vi "Example - Creating and Building an Installer.vi"() -> ()   [LabVIEW 2020]
doc: "Demonstrates the use of the Installer Builder API to create and build an Installer build specification."
uses:
  <vilib>/InstallerBuilder/Classes/Win_Installer/Product Version.ctl
  <vilib>/InstallerBuilder/Classes/Win_Installer/AB_Win_Installer.lvclass/AB_Win_Installer.ctl
  <vilib>/InstallerBuilder/Classes/Win_Source/AB_Win_Source.lvclass/AB_Win_Source.ctl
  <vilib>/InstallerBuilder/Classes/Win_Source/Get Name.vi
  <vilib>/InstallerBuilder/Classes/Win_Source/Get Install Path.vi
  <vilib>/InstallerBuilder/Classes/Win_Installer/Set Auto-increment Version.vi
  <vilib>/InstallerBuilder/Classes/Win_Installer/Set Product Version.vi
  <vilib>/InstallerBuilder/Classes/Win_Installer/Get Default Install Directory.vi
  <vilib>/InstallerBuilder/Classes/Win_Source_File/AB_Win_Source_File.lvclass
  e:/builds/penguin/labview/branches/2020/dev/dist/vi.lib/InstallerBuilder/Classes/Win_Source/AB_Win_Source.lvclass
  <vilib>/InstallerBuilder/Classes/Win_Installer/Get Installed Files.vi
  <vilib>/InstallerBuilder/Classes/Win_Installer/Get System Folder (Desktop).vi
  <vilib>/AppBuilder/AB_API_Simple/Build (project reference).vi
  <vilib>/InstallerBuilder/Classes/Win_Installer/AB_Win_Installer.lvclass
  <vilib>/AppBuilder/AB_API_Simple/NI_App_Builder_API.lvlib
panel:
  out "Files included in the installer":string[](array[string])
  # "Overview: Demonstrates the use of the Installer Builder API to create and build an Installer build specification.\nRequirements: LabVIEW Professional Development System or LabVIEW Application Builder\nInstructions:\n1. Run the VI. An Installer build specification will be created, which will then be built programmatically.\n2. A project window will open. Examine the New Installer build specification in the new project.\n3. Close the temporary project and delete the temporary project files generated by this example when you are done.\n4. In the Project Explorer window, right-click on the New Installer build specification and choose Explore to navigate to the installer and run it."
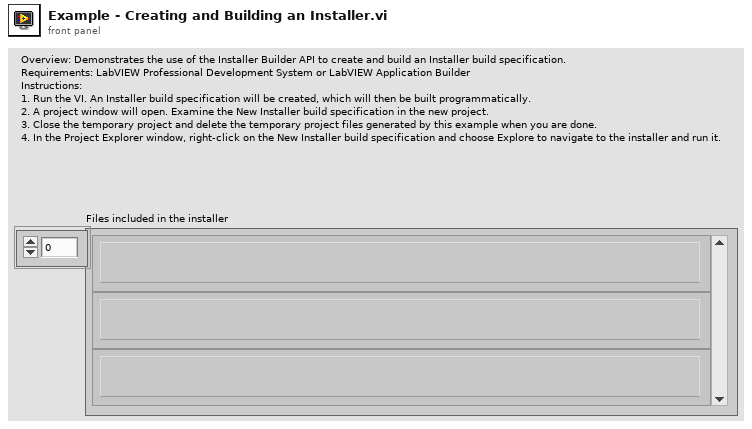
[diagram p1: front panel]
types:
  T1 = typedef "AB_Win_Installer.lvclass/Product Version.ctl" = cluster{"Major":u8, "Minor":u8, "Update":u16}
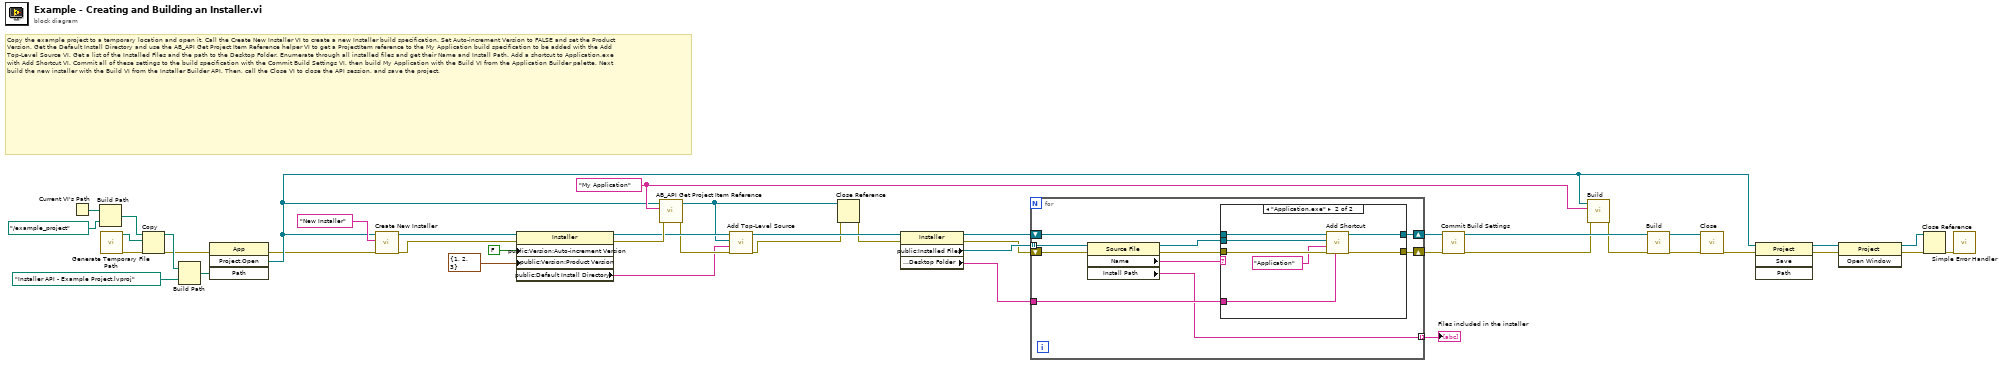
[diagram p0: block diagram]
diagram:
  w15 = "My Application" ("Name")
  # "Copy the example project to a temporary location and open it. Call the Create New Installer VI to create a new Installer build specification. Set Auto-increment Version to FALSE and set the Product Version. Get the Default Install Directory and use the AB_API Get Project Item Reference helper VI to get a ProjectItem reference to the My Application build specification to be added with the Add Top-Level Source VI. Get a list of the Installed Files and the path to the Desktop Folder. Enumerate through all installed files and get their Name and Install Path. Add a shortcut to Application.exe with Add Shortcut VI. Commit all of these settings to the build specification with the Commit Build Settings VI, then build My Application with the Build VI from the Application Builder palette. Next build the new installer with the Build VI from the Installer Builder API. Then, call the Close VI to close the API session, and save the project."
  n1 = Current VI's Path() -> (path=w43:path)
  n2 = Build Path(base path=w43, name or relative path=path "../example_project" ("path")) -> (appended path=w41:path)
  n3 = call <vilib>:"Generate Temporary File Path.vi"() -> ("error out"=w35:errorcluster, "Unique Temporary File Path"=w40:path)  [unwired: 10 in]
  n4 = Copy(8:w35, 10:w40, 11:w41) -> (0:w34:errorcluster, 3:w39:path)  [unwired: 2 in, 1 out]
  n5 = Build Path(base path=w39, name or relative path=path "Installer API - Example Project.lvproj") -> (appended path=w37:path)
  n6 = invoke class="App" method="Project.Open"(error in=w34, "Path"=w37) -> (error out=w8:errorcluster, "Project:Open"=w9:refnum<vi>)  [unwired: 2 in, 2 out]
  n7 = call <vilib>:"Create New Installer.vi"("error in (no error)"=w8, "Build Specification Name"="New Installer", "Project Refnum"=w9) -> ("error out"=w28:errorcluster, "AB_Win_Installer out"=w30:refnum<class "AB_Win_Installer.lvclass">)  [unwired: 7 in]
  n8 = property class="Installer"(reference=w30, error in=w28, "public:Version:Auto-increment Version"=FALSE ("Version:Auto-increment Version"), "public:Version:Product Version"=T1 {"Major"=1, "Minor"=2, "Update"=3} ("Version:Product Version")) -> (reference out=w24:refnum<class "AB_Win_Installer.lvclass">, error out=w25:errorcluster, "public:Default Install Directory"=w22:string)
  n9 = call <vilib>:"AB_API Get Project Item Reference.vi"("error in (no error)"=w25, "Name"=w15, "Project Refnum"=w9) -> ("error out"=w23:errorcluster, "ProjectItem Refnum"=w3:refnum<vi>)  [unwired: 6 in, 1 out]
  n10 = call <vilib>:"Add Top-Level Source.vi"("error in (no error)"=w23, "Install Path"=w22, "ProjectItem Refnum"=w3, "AB_Win_Installer in"=w24) -> ("error out"=w2:errorcluster, "AB_Win_Installer out"=w20:refnum<class "AB_Win_Installer.lvclass">)  [unwired: 5 in, 1 out]
  n11 = Close Reference(reference=w3, error in (no error)=w2) -> (error out=w1:errorcluster)
  n12 = property class="Installer"(reference=w20, error in=w1) -> (reference out=w12:refnum<class "AB_Win_Installer.lvclass">, error out=w17:errorcluster, "public:Installed Files"=w19:refnum<class "AB_Win_Source_File.lvclass">[], "public:System Paths:Desktop Folder"=w10:string)
  n13 = for {
    tunnel: w19 -> [w53] mode=indexing
    shift-right: [w46] -> w16
    shift-left: w17 -> [w52]
    tunnel: [w44] -> w18 mode=indexing
    shift-right: [w50] -> w11
    shift-left: w12 -> [w51]
    tunnel: w10 -> [w48]
    n14 = property class="Source File"(reference=w53, error in=w52) -> (reference out=w49:refnum<class "AB_Win_Source_File.lvclass">, error out=w47:errorcluster, "Name"=w45:string, "Install Path"=w44:string)
    n15 = case shown="\"Application.exe\"" w45 {
      tunnel: w51 -> [w55 w62]
      tunnel: [w55 w60] -> w50
      tunnel: w49 -> [_ w61]
      tunnel: w48 -> [_ w59]
      tunnel: w47 -> [w54 w58]
      tunnel: [w54 w57] -> w46
      frame Default {
      }
      frame "Application.exe" {
        n16 = call <vilib>:"Add Shortcut.vi"("Shortcut Path"=w59, "error in (no error)"=w58, "Shortcut Name"="Application", "Source File"=w61, "AB_Win_Installer in"=w62) -> ("error out"=w57:errorcluster, "AB_Win_Installer out"=w60:refnum<class "AB_Win_Installer.lvclass">)  [unwired: 4 in, 1 out]
      }
    }
  }
  "Files included in the installer" <- w18
  n17 = call <vilib>:"Commit Build Settings.vi"("error in (no error)"=w16, "AB_Win_Installer in"=w11) -> ("error out"=w14:errorcluster, "AB_Win_Installer out"=w31:refnum<class "AB_Win_Installer.lvclass">)  [unwired: 8 in]
  n18 = call-poly <vilib>:"Build.vi"("error in (no error)"=w14, "Name of build specification (if empty: build all)"=w15, "Project reference"=w9) -> ("error out"=w13:errorcluster)  [unwired: 6 in, 2 out]
  n19 = call <vilib>:"Build.vi"("error in (no error)"=w13, "AB_Win_Installer in"=w31) -> ("error out"=w32:errorcluster, "AB_Win_Installer out"=w33:refnum<class "AB_Win_Installer.lvclass">)  [unwired: 8 in]
  n20 = call <vilib>:"Close.vi"("error in (no error)"=w32, "AB_Win_Installer in"=w33) -> ("error out"=w21:errorcluster)  [unwired: 9 in]
  n21 = invoke class="Project" method="Save"(reference=w9, error in=w21) -> (reference out=w7:refnum<vi>, error out=w5:errorcluster)  [unwired: 2 in, 2 out]
  n22 = invoke class="Project" method="Open Window"(reference=w7, error in=w5) -> (reference out=w6:refnum<vi>, error out=w4:errorcluster)  [unwired: 1 in, 1 out]
  n23 = Close Reference(reference=w6, error in (no error)=w4) -> (error out=w42:errorcluster)
  n24 = call <vilib>:"Simple Error Handler.vi"("error in (no error)"=w42) -> ()  [unwired: 4 in, 5 out]
